vi "Create Data Store.vi"(8 "error in (no error)":errorcluster, 11 "Scan Driver.lvclass in":refnum<class "Scan Driver.lvclass">) -> (0 "error out":errorcluster, 3 "Scan Driver.lvclass out":refnum<class "Scan Driver.lvclass">)   [LabVIEW 2017, in "Scan Driver.lvclass"]
doc: "Initialize the internal Data Store. Call member Scanner instance to do the same."
uses:
  Scan Driver.lvclass
  Scanners/Scanner/Scanner.lvclass
  Readers/Reader/Reader.lvclass
  Data Processing/Aux Data Source/Aux Data Source.lvclass
  Instruments/Utility Classes/Readable/Data Point.ctl
  Instruments/Utility Classes/Readable/Readable.lvclass
  Instruments/Utility Classes/Readable/Data Channel.ctl
  Instruments/Utility Classes/Readable/X.ctl
  Instruments/Utility Classes/Readable/Time.ctl
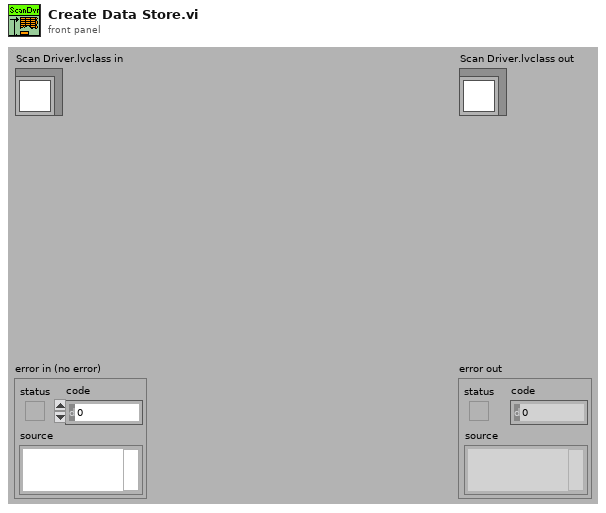
[diagram p1: front panel]
types:
  T1 = typedef "Readable.lvclass/Data Channel.ctl" = cluster{"Name":string, "Data Point":T2, "Unit":string}
  T2 = typedef "Readable.lvclass/Data Point.ctl" = cluster{"t":T3, "x":T4}
  T3 = typedef "Readable.lvclass/Time.ctl" = timestamp
  T4 = typedef "Readable.lvclass/X.ctl" = dbl
  T5 = typedef "Readable.lvclass/Data Channels.ctl" = T1[]
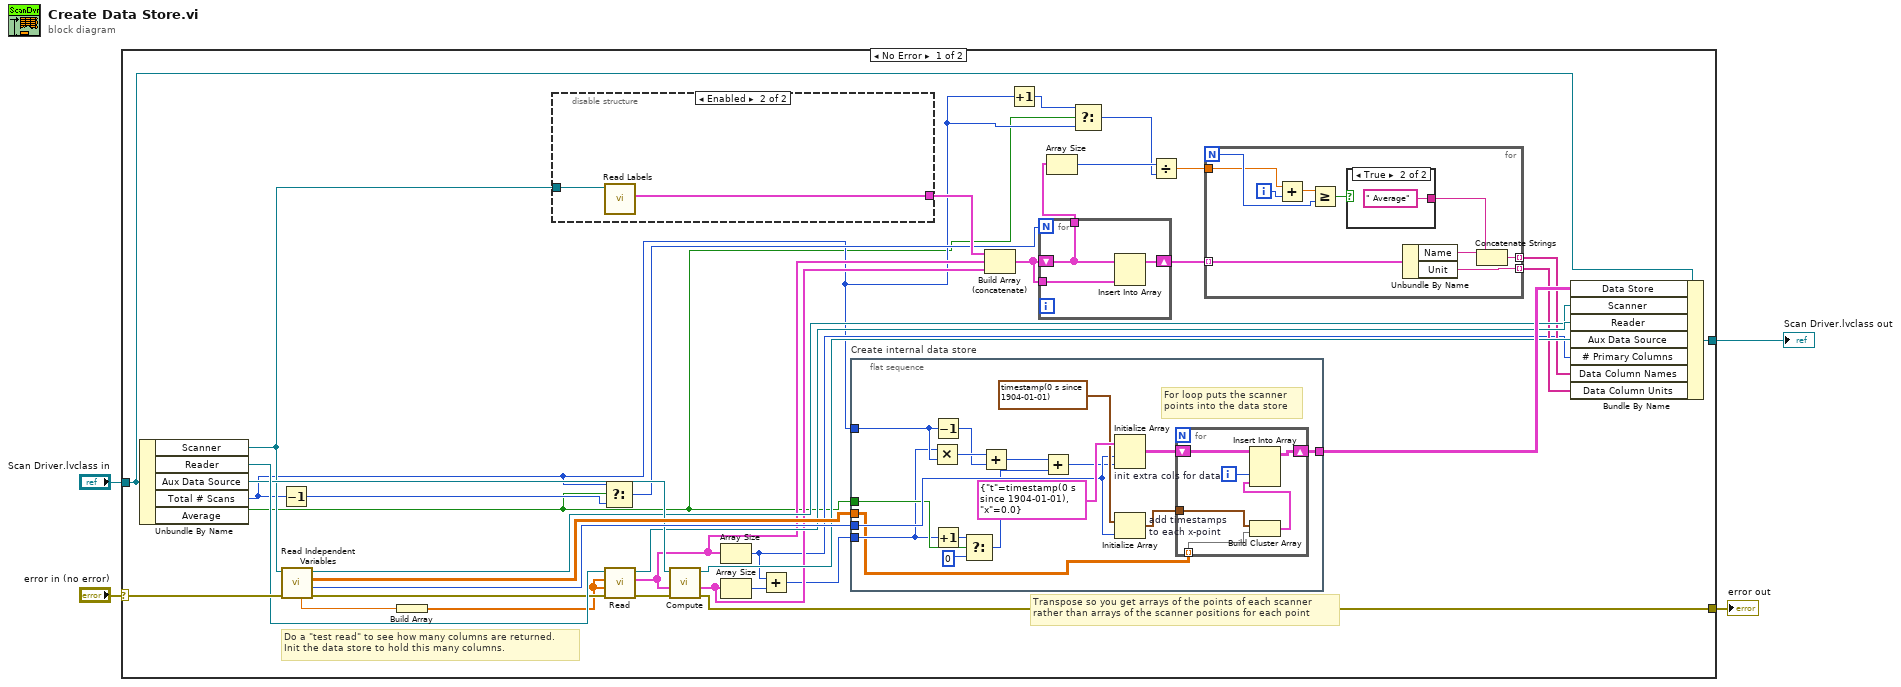
[diagram p0: block diagram]
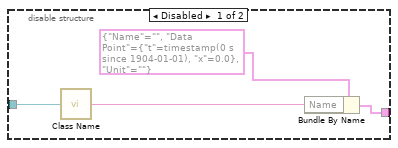
[diagram p2: hidden frame]
diagram:
  n1 = case shown="No Error" "error in (no error)" {
    selector: "error in (no error)" -> [w35 w84]
    tunnel: [w27 w84] -> w3
    tunnel: [w40 w85] -> w1
    tunnel: "Scan Driver.lvclass in" -> [w37 w85]
    frame No Error {
      # "Transpose so you get arrays of the points of each scanner \nrather than arrays of the scanner positions for each point"
      # "Do a \"test read\" to see how many columns are returned.\nInit the data store to hold this many columns."
      n2 = Unbundle By Name(w37) -> ("Scanner"=w20:refnum<class "Scanner.lvclass">, "Reader"=w34:refnum<class "Reader.lvclass">, "Aux Data Source"=w33:refnum<class "Aux Data Source.lvclass">, "Total # Scans"=w10:u32, "Average"=w7:bool)
      n3 = Decrement(x=w10) -> (x-1=w15:u32)
      n4 = call-dynamic "Read Independent Variables.vi"("error in (no error)"=w35, "Scanner.lvclass in"=w20) -> ("error out"=w29:errorcluster, "size"=w36:i32, "Independent Variables"=w38:dbl[][], "Scanner.lvclass out"=w26:refnum<class "Scanner.lvclass">, "min value"=w6:dbl)  [unwired: 5 out]
      n5 = Build Array(w6) -> (w5:dbl[])
      n6 = disable-structure shown="Enabled" {
        disable-tunnel: [w46 w48] -> w21
        disable-tunnel: w20 -> [w45 w49]
        frame Disabled {
          n7 = call "Class Name.vi"("LabVIEW Object"=w45) -> ("Classname"=w44:string)
          n8 = Bundle By Name(cluster=T1 {"Name"="", "Data Point"={"t"=timestamp(0 s since 1904-01-01), "x"=0.0}, "Unit"=""} ("Add'l Data Channels"), "Name"=w44) -> (w46:T1)
        }
        frame Enabled {
          n9 = call-dynamic "Read Labels.vi"("Scanner in"=w49) -> ("Axis Label and Unit"=w48:T1[])  [unwired: 8 in, 2 out]
        }
      }
      n10 = Select(t=w10, s=w7, f=w15) -> (s? t:f=w17:u32)
      n11 = call-dynamic "Read.vi"("error in (no error)"=w29, "Starting independent variables"=w5, "Current independent variables"=w5, "Reader in"=w34) -> ("error out"=w30:errorcluster, "Data Channels"=w24:T5, "Reader out"=w32:refnum<class "Reader.lvclass">)  [unwired: 5 in]
      n12 = call-dynamic "Compute.vi"("error in (no error)"=w30, "Data Channels"=w24, "Aux Data Source in"=w33) -> ("error out"=w27:errorcluster, "Add'l Data Channels"=w25:T5, "Aux Data Source out"=w31:refnum<class "Aux Data Source.lvclass">)  [unwired: 6 in]
      n13 = Array Size(array=w24) -> (size(s)=w14:i32)
      n14 = Array Size(array=w25) -> (size(s)=w28:i32)
      n15 = Add(x=w14, y=w28) -> (x+y=w19:i32)
      n16 = flat-sequence "Create internal data store" {
        tunnel: [w62] -> w39
        tunnel: w38 -> [w61]
        tunnel: w36 -> [w75]
        tunnel: w19 -> [w68]
        tunnel: w10 -> [w73]
        tunnel: w7 -> [w72]
        frame #0 {
          # "For loop puts the scanner \npoints into the data store"
          n17 = Multiply(x=w68, y=w73) -> (x*y=w74:u32)
          n18 = Decrement(x=w73) -> (x-1=w70:u32)
          n19 = Increment(x=w68) -> (x+1=w67:i32)
          n20 = Select(t=w67, s=w72, f=0 ("index (row)")) -> (s? t:f=w65:i32)
          n21 = Add(x=w74, y=w70) -> (x+y=w69:u32)
          n22 = Add(x=w69, y=w65) -> (x+y=w66:u32)
          n23 = Initialize Array "init extra cols for data"(T2 {"t"=timestamp(0 s since 1904-01-01), "x"=0.0}, w75, w66) -> (w64:T2[][])
          n24 = Initialize Array "add timestamps\nto each x-point"(T3 timestamp(0 s since 1904-01-01) ("t"), w75) -> (w63:T3[])
          n25 = for {
            tunnel: w63 -> [w81]
            tunnel: w61 -> [w80] mode=indexing
            shift-right: [w78] -> w62
            shift-left: w64 -> [w82]
            i -> [w79]
            n26 = Build Cluster Array(w81, w80) -> (w83:cluster{"t":T3, "Numeric":dbl}[])
            n27 = Insert Into Array(array=w82, index (col)=w79, new element=w83) -> (w78:T2[][])  [unwired: 1 in]
          }
        }
      }
      n28 = Build Array (concatenate)(w21, w24, w25) -> (w18:T5)
      n29 = Increment(x=w10) -> (x+1=w11:u32)
      n30 = for {
        N: w17 -> [_]
        shift-right: [w42] -> w16
        shift-left: w18 -> [w41]
        tunnel: w18 -> [w43]
        tunnel: [w41] -> w9
        n31 = Insert Into Array(array=w41, new element=w43) -> (w42:T5)  [unwired: 1 in]
      }
      n32 = Array Size(array=w9) -> (size(s)=w13:i32)
      n33 = Select(t=w11, s=w7, f=w10) -> (s? t:f=w12:u32)
      n34 = Divide(x=w13, y=w12) -> (x/y=w8:dbl)
      n35 = for {
        N -> [w53]
        tunnel: w16 -> [w59] mode=indexing
        tunnel: [w52] -> w23 mode=indexing
        tunnel: [w57] -> w22 mode=indexing
        tunnel: w8 -> [w50]
        i -> [w54]
        n36 = Add(x=w50, y=w54) -> (x+y=w55:dbl)
        n37 = Greater Or Equal?(x=w55, y=w53) -> (x >= y?=w56:bool)
        n38 = case shown="True" w56 {
          tunnel: [_ " Average"] -> w51
          frame False {
          }
          frame True {
          }
        }
        n39 = Unbundle By Name(w59) -> ("Name"=w58:string, "Unit"=w57:string)
        n40 = Concatenate Strings(w58, w51) -> (w52:string)
      }
      n41 = Bundle By Name(cluster=w37, "Data Store"=w39, "Scanner"=w26, "Reader"=w32, "Aux Data Source"=w31, "# Primary Columns"=w14, "Data Column Names"=w23, "Data Column Units"=w22) -> (w40:refnum<class "Scan Driver.lvclass">)
    }
    frame Error {
    }
  }
  "error out" <- w3
  "Scan Driver.lvclass out" <- w1
